vi "Parse Bitfile for EST IP.vi"(8 "error in (no error)":errorcluster, 10 "bitfile path":path, 11 "Item Ref in":T1 format="%.0x") -> (0 "error out":errorcluster, 1 "APUs":string[](array[string]), 2 "version":string, 3 "Item Ref out":T1 format="%.0x")   [LabVIEW 2013, in "Engine Simulation Toolkit System Explorer.lvlib"]
uses:
  Engine Simulation Toolkit System Explorer.lvlib
  <vilib>/NI Veristand/Custom Device API/Custom Device Item Ref.ctl
  Shared/Properties.vi
  <vilib>/NI Veristand/Custom Device API/Set Item Property (Boolean).vi
  Shared/Constants and GUIDs.vi
  <vilib>/NI Veristand/Custom Device API/Set Item Property (String).vi
  <vilib>/NI Veristand/Custom Device API/Custom Device API.lvlib
  Shared/Engine Simulation Toolkit Shared.lvlib
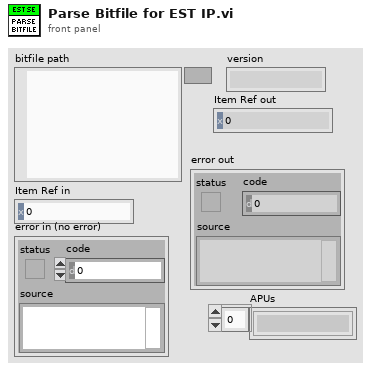
[diagram p1: front panel]
types:
  T1 = typedef "Custom Device API.lvlib/Custom Device Item Ref.ctl" = u64
  T2 = typedef "Engine Simulation Toolkit Shared.lvlib/Bitfile EST Version.ctl" = enum16{"1.0", "1.1", "1.2", "1.3"}
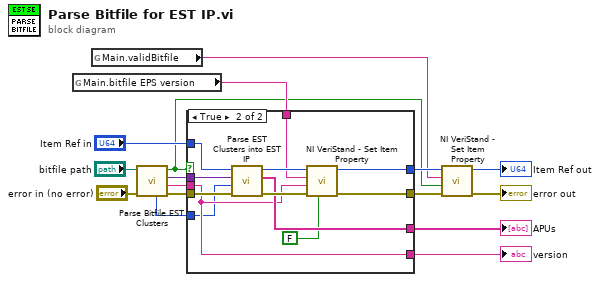
[diagram p0: block diagram]
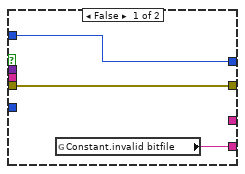
[diagram p2: hidden frame]
diagram:
  n1 = global read "Properties.vi" "Main.bitfile EPS version"() -> (w12:string)
  n2 = global read "Properties.vi" "Main.validBitfile"() -> (w4:string)
  n3 = call "Parse Bitfile EST Clusters.vi"("error in (no error)"="error in (no error)", "bitfile path"="bitfile path") -> ("error out"=w16:errorcluster, "version"=w11:string, "EPS IP LUT"=w14:variant, "valid bitfile"=w3:bool, "EST version enum"=w1:T2)  [unwired: 5 in]
  n4 = case shown="True" w3 {
    tunnel: w16 -> [w19 w31]
    tunnel: w14 -> [_ w30]
    tunnel: "Item Ref in" -> [w18 w29]
    tunnel: w12 -> [_ w26]
    tunnel: w11 -> [_ w22]
    tunnel: [w19 w25] -> w9
    tunnel: [w18 w24] -> w6
    tunnel: [_ w23] -> w8
    tunnel: [w17 w22] -> w2
    tunnel: w1 -> [_ w21]
    frame False {
      n5 = global read "Constants and GUIDs.vi" "Constant.invalid bitfile"() -> (w17:string)
    }
    frame True {
      n6 = call "Parse EST Clusters into EST IP.vi"("error in (no error)"=w31, "EST version enum"=w21, "EPS IP LUT"=w30, "Item Ref in"=w29) -> ("error out"=w27:errorcluster, "APUs"=w23:string[], "Item Ref out"=w28:T1)  [unwired: 5 in]
      n7 = call-poly <vilib>:"NI VeriStand - Set Item Property.vi"("Binary String (T)"=FALSE, "error in (no error)"=w27, "Value"=w22, "Property Name"=w26, "Item Ref in"=w28) -> ("error out"=w25:errorcluster, "Item Ref out"=w24:T1)  [unwired: 4 in, 1 out]
    }
  }
  "version" <- w2
  "APUs" <- w8
  n8 = call-poly <vilib>:"NI VeriStand - Set Item Property.vi"("error in (no error)"=w9, "Value"=w3, "Property Name"=w4, "Item Ref in"=w6) -> ("error out"=→"error out":errorcluster, "Item Ref out"=→"Item Ref out":T1)  [unwired: 5 in, 1 out]
